vi "MainBancoEiettori.vi"() -> ()   [LabVIEW 2025]
uses:
  STATES_MACHINE.ctl
  <instrlib>/Bronkhorst FLOW-BUS/Public/Configure/Setpoint/Configure Setpoint (Direct).vi
  <instrlib>/Bronkhorst FLOW-BUS/Public/Data/Measure/Read Measure (Direct).vi
  <vilib>/Utility/file.llb/Write Delimited Spreadsheet (string).vi
  <vilib>/Utility/file.llb/Write Delimited Spreadsheet (DBL).vi
  <instrlib>/Bronkhorst FLOW-BUS/Bronkhorst FLOW-BUS.lvlib
panel:
  in  "Tab Control":enum32{"Main", "Debug"}(tab)
  in  "Sample Time":u16=100
  in  "Clear Graph":bool
  in  "Start Test Session":bool
  in  "stop":bool
  out "array":dbl[][](array[numeric]) format="%#_5g"
  out "Outlet  [mA]":dbl
  out "Secondary [mA]":dbl
  out "Primary [mA]":dbl
  out "Outlet [bar]":dbl
  out "Secondary [bar]":dbl
  out "Primary [bar]":dbl
  in  "Insert Case":bool
  in  "New test":bool
  out "Waveform Chart":T1(graph)
  out "Exit":bool
  out "_InsertCase":bool
  out "_NewTest":bool
  in  "VISA resource name 2":refnum<visa-resource-name>
  out "Fluid Name":string
  out "Capacity":sgl
  out "Capacity Unit":string
  out "Capacity Unit 2":string
  out "Capacity 2":sgl
  out "Fluid Name 2":string
  in  "VISA resource name 3":refnum<visa-resource-name>
  out "_StartSession":bool
  # "Current \nValve\n[mA]"
  # "Primary \nPressure\n[bar]"
  # "Secondary \nPressure\n[bar]"
  # "Outlet \nPressure\n[bar]"
  # "Mass Flow\nPrimary\nkg/min"
  # "Mass Flow\nSecondary\nkg/min"
  # "Actual Pressure Values"
  # "ms"
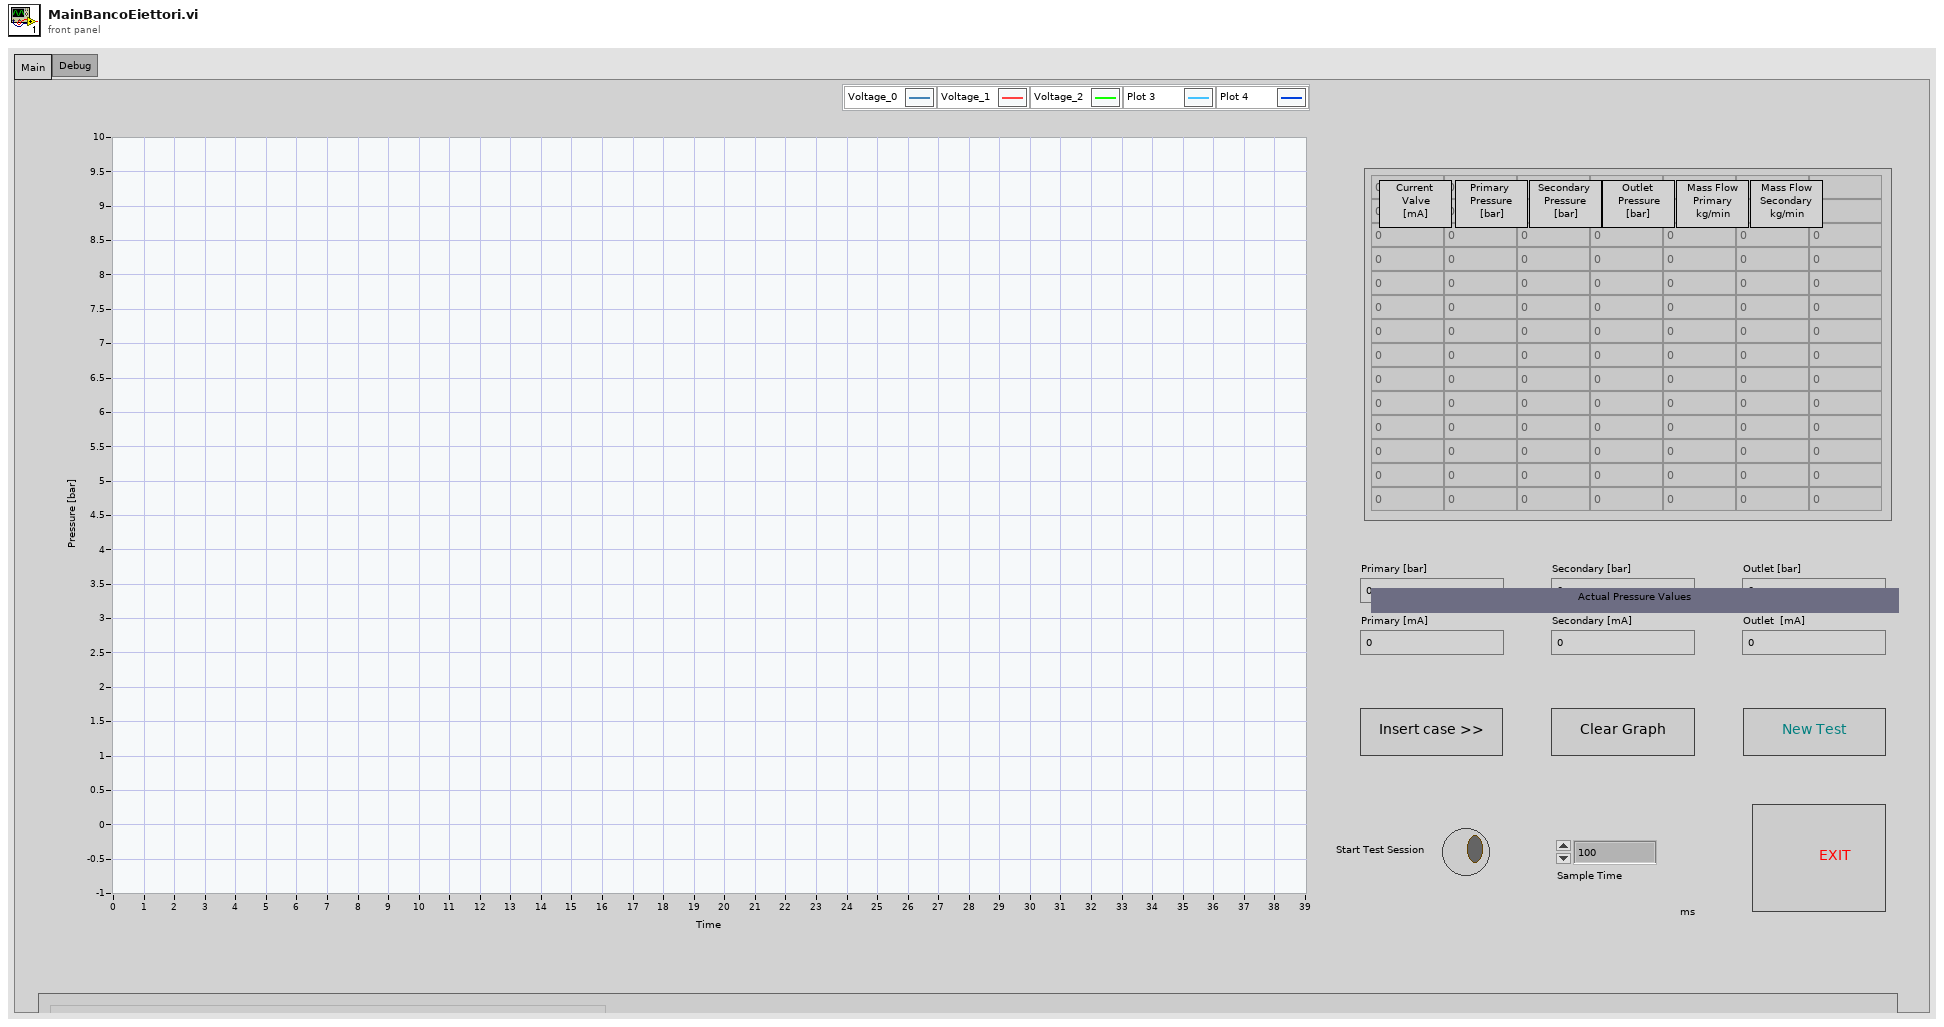
[diagram p1: front panel]
types:
  T1 = cluster{"Scalar":dbl, "Scalar":dbl, "Scalar":dbl, "number: 0 to 1":dbl, "number: 0 to 1":dbl}
  T2 = typedef "STATES_MACHINE.ctl" = enum16{"INIT", "TEST", "CLOSE"}
  T3 = cluster{"Scalar":dbl, "Scalar":dbl, "Scalar":dbl, "number: 0 to 1":dbl, "number: 0 to 1":dbl}[]
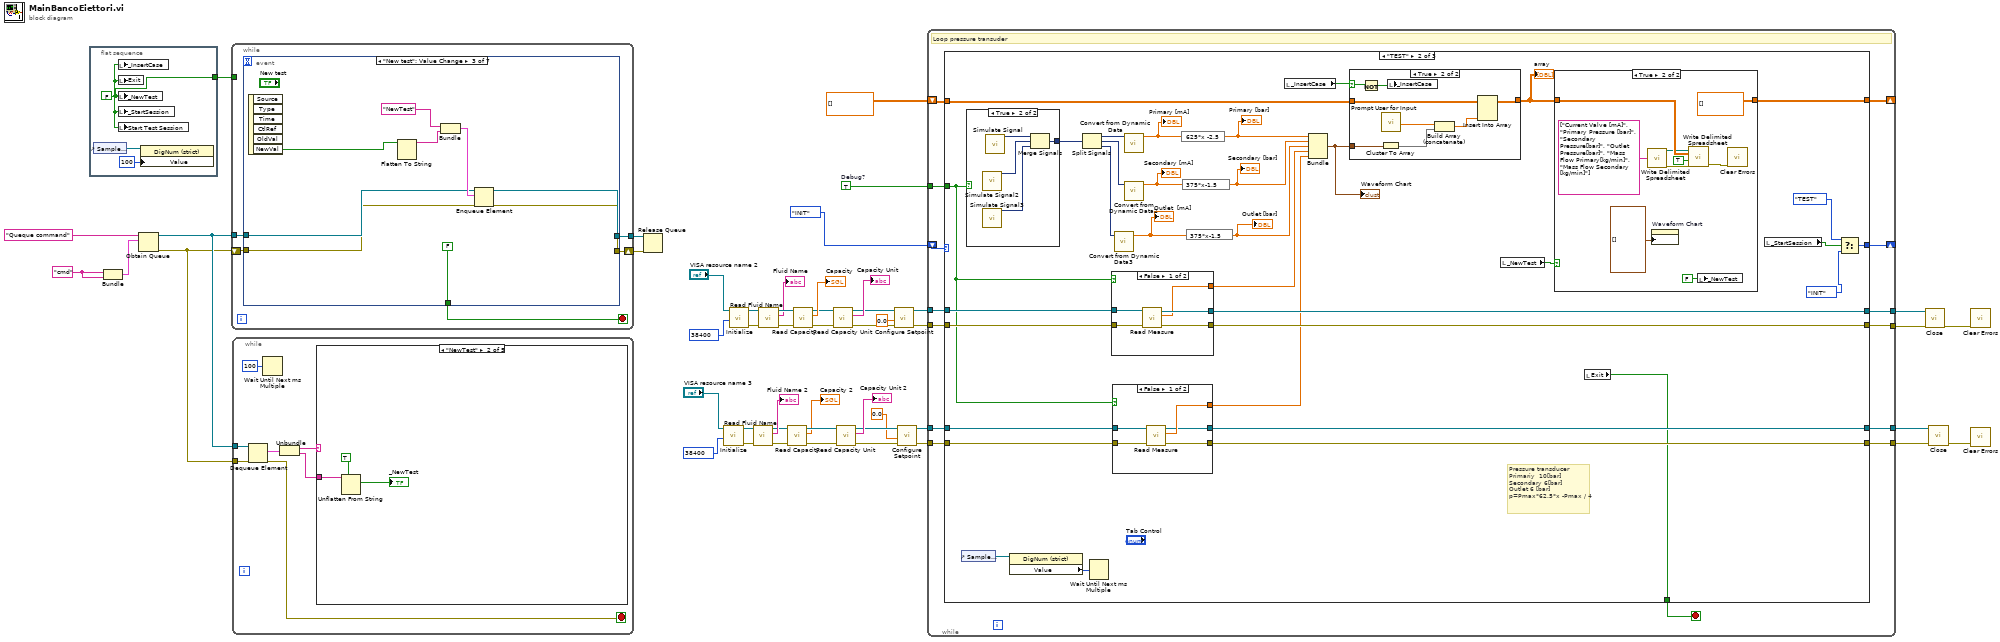
[diagram p0: block diagram]
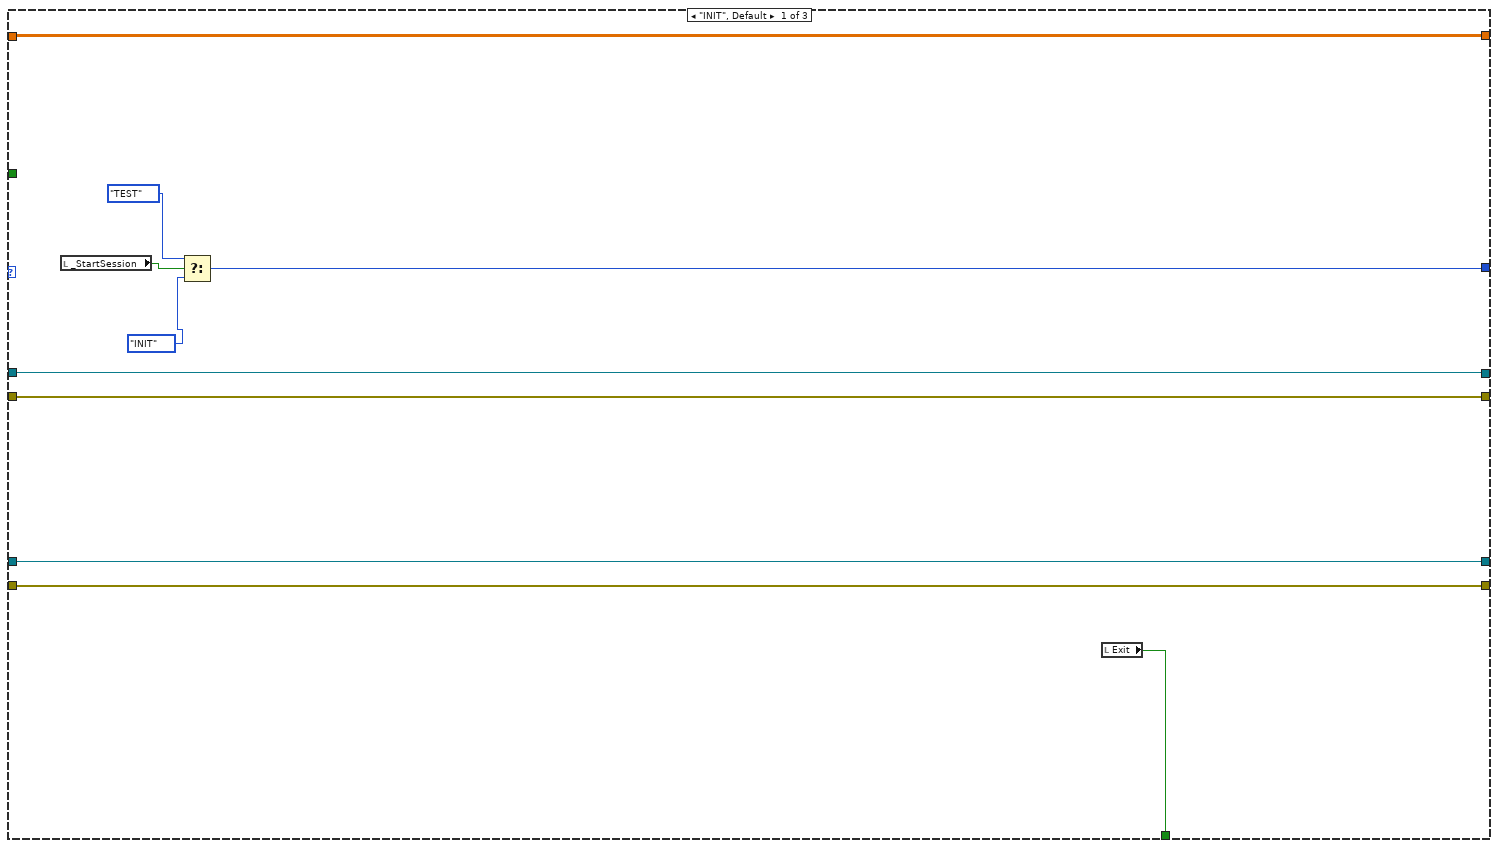
[diagram p2: hidden frame]
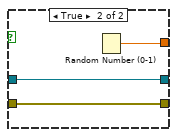
[diagram p3: hidden frame]
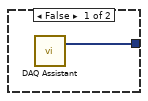
[diagram p4: hidden frame]
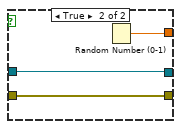
[diagram p7: hidden frame]
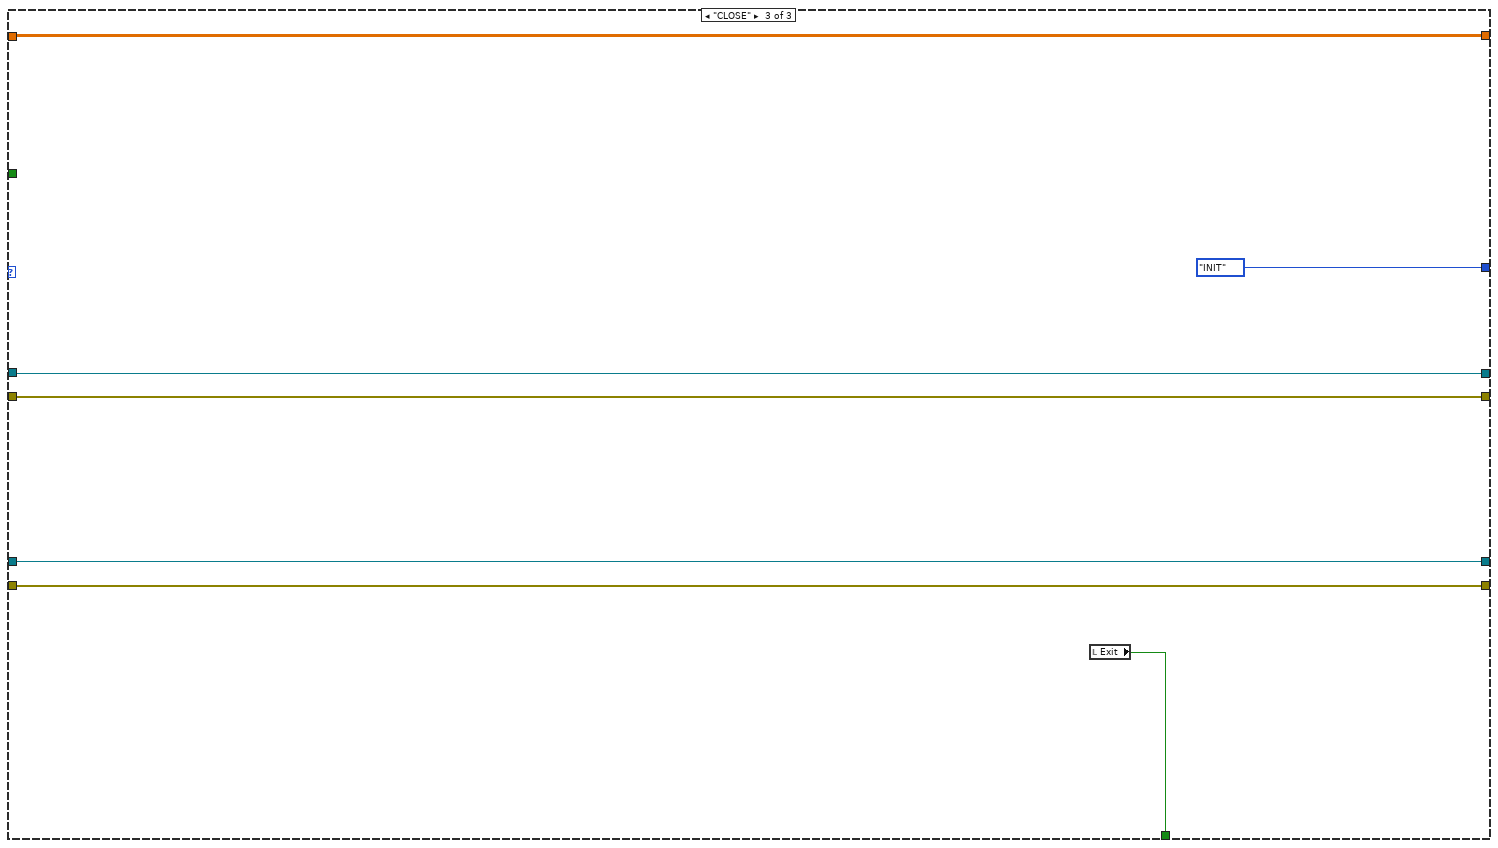
[diagram p8: hidden frame]
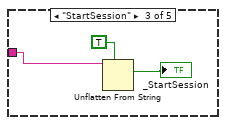
[diagram p10: hidden frame]
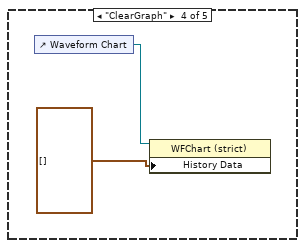
[diagram p11: hidden frame]
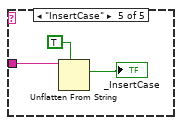
[diagram p12: hidden frame]
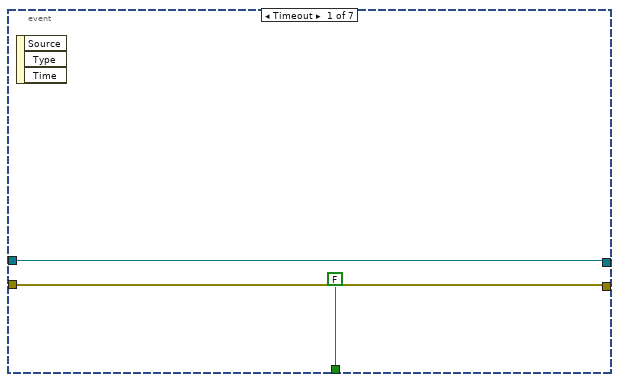
[diagram p13: hidden frame]
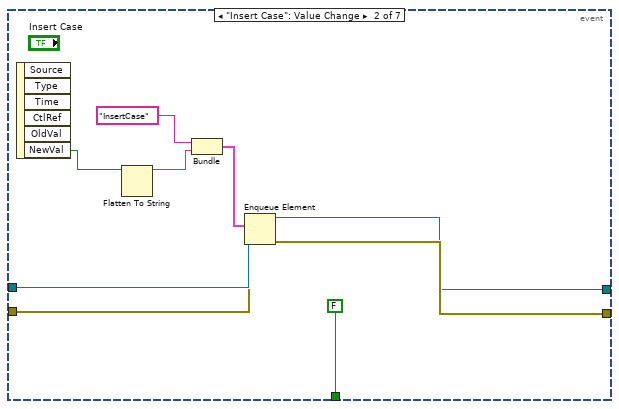
[diagram p14: hidden frame]
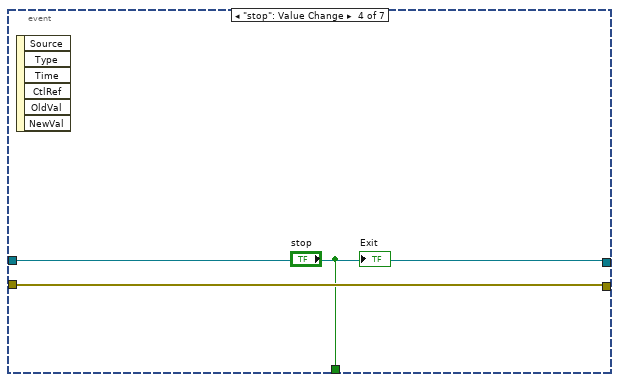
[diagram p15: hidden frame]
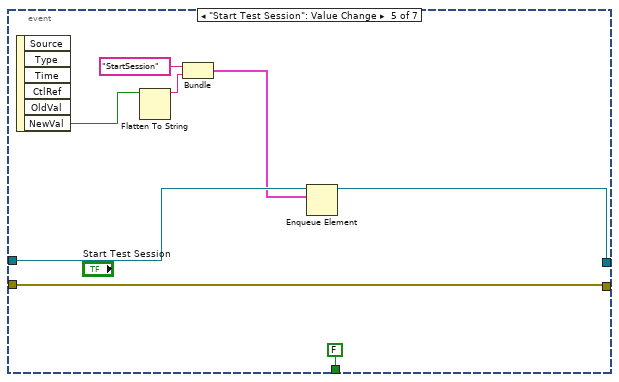
[diagram p16: hidden frame]
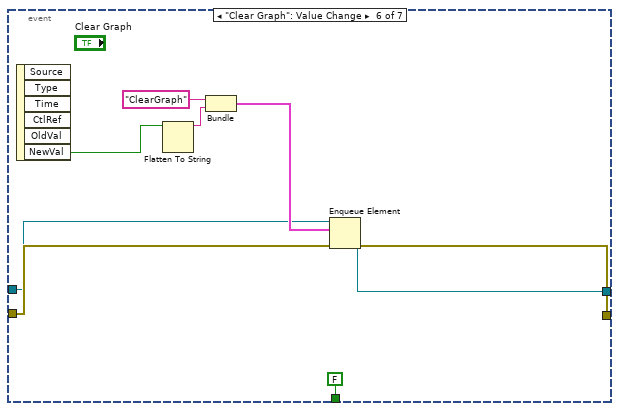
[diagram p17: hidden frame]
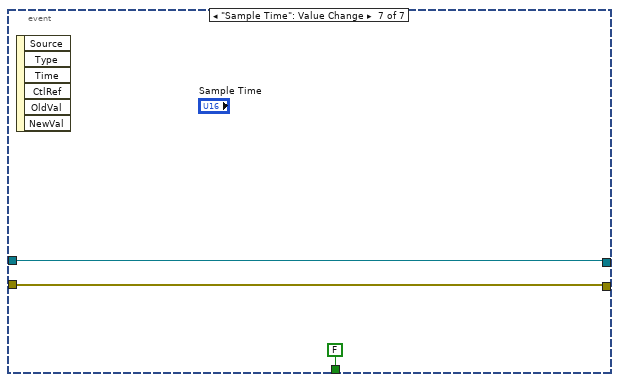
[diagram p18: hidden frame]
diagram:
  w13 = TRUE  # Debug?
  w27 = u32 38400 items=["9600"=9600, "19200"=19200, "38400"=38400, "57600"=57600, "115200"=115200, "230400"=230400, "460800"=460800] ("Baud Rate (38400)")
  w32 = u32 38400 items=["9600"=9600, "19200"=19200, "38400"=38400, "57600"=57600, "115200"=115200, "230400"=230400, "460800"=460800] ("Baud Rate (38400)")
  w42 = "cmd"
  n1 = flat-sequence {
    tunnel: [w52] -> w41
    frame #0 {
      w52 = FALSE ("_InsertCase 2")
      n2 = control-ref of="Sample Time"() -> (w51:refnum<vi>)
      n3 = local write "_InsertCase"(w52) -> ()
      n4 = local write "Exit"(w52) -> ()
      n5 = local write "_NewTest"(w52) -> ()
      n6 = local write "_StartSession"(w52) -> ()
      n7 = local write "Start Test Session"(w52) -> ()
      n8 = property class="DigNum (strict)"(reference=w51, "Value"=u16 100) -> ()  [unwired: 1 in, 2 out]
    }
  }
  n9 = Bundle(w42, w42) -> (w47:cluster{string, string})  [unwired: 1 in]
  n10 = Obtain Queue(name (unnamed)="Queque command", element data type=w47) -> (queue out=w44:refnum<queue>, error out=w43:errorcluster)  [unwired: 3 in, 1 out]
  n11 = while {
    tunnel: w44 -> [w57]
    shift-right: [w55] -> w45
    shift-left: w43 -> [w56]
    tunnel: [w54] -> w46
    tunnel: w41 -> [_]
    stop <- w53 stop-if-true
    n12 = event shown="[2] \"New test\": Value Change" {
      selector: _ -> [_ _ _ _ _ _ _]
      dyn-events: _ -> [_ _ _ _ _ _ _]
      timeout: _ -> [_ _ _ _ _ _ _]
      tunnel: w57 -> [w60 w69 w74 w81 w88 w92 w100]
      tunnel: w56 -> [w59 w68 w73 w80 w89 w95 w101]
      tunnel: [w59 w67 w71 w80 w89 w94 w101] -> w55
      tunnel: [w60 w66 w72 w81 w87 w93 w100] -> w54
      tunnel: [FALSE ("stop") FALSE ("stop") FALSE ("stop") "stop" FALSE ("stop") FALSE ("stop") FALSE ("stop")] -> w53
      event Timeout {
        n13 = event-data() -> ()  [unwired: 1 in, 3 out]
      }
      event "Insert Case": Value Change {
        n14 = event-data() -> ("NewVal"=w61:bool)  [unwired: 1 in, 5 out]
        n15 = Flatten To String(anything=w61) -> (data string=w64:string)  [unwired: 3 in, 2 out]
        n16 = Bundle("InsertCase", "data string"=w64) -> (w63:cluster{string, "data string":string})  [unwired: 1 in]
        n17 = Enqueue Element(queue=w69, element=w63, error in (no error)=w68) -> (queue out=w66:refnum<queue>, error out=w67:errorcluster)  [unwired: 1 in, 1 out]
      }
      event "New test": Value Change {
        n18 = event-data() -> ("NewVal"=w70:bool)  [unwired: 1 in, 5 out]
        n19 = Flatten To String(anything=w70) -> (data string=w76:string)  [unwired: 3 in, 2 out]
        n20 = Bundle("NewTest", "data string"=w76) -> (w75:cluster{string, "data string":string})  [unwired: 1 in]
        n21 = Enqueue Element(queue=w74, element=w75, error in (no error)=w73) -> (queue out=w72:refnum<queue>, error out=w71:errorcluster)  [unwired: 1 in, 1 out]
      }
      event "stop": Value Change {
        n22 = event-data() -> ()  [unwired: 1 in, 6 out]
        "Exit" <- "stop"
      }
      event "Start Test Session": Value Change {
        n23 = event-data() -> ("NewVal"=w85:bool)  [unwired: 1 in, 5 out]
        n24 = Flatten To String(anything=w85) -> (data string=w84:string)  [unwired: 3 in, 2 out]
        n25 = Bundle("StartSession", "data string"=w84) -> (w83:cluster{string, "data string":string})  [unwired: 1 in]
        n26 = Enqueue Element(queue=w88, element=w83) -> (queue out=w87:refnum<queue>)  [unwired: 2 in, 2 out]
      }
      event "Clear Graph": Value Change {
        n27 = event-data() -> ("NewVal"=w91:bool)  [unwired: 1 in, 5 out]
        n28 = Flatten To String(anything=w91) -> (data string=w97:string)  [unwired: 3 in, 2 out]
        n29 = Bundle("ClearGraph", "data string"=w97) -> (w96:cluster{string, "data string":string})  [unwired: 1 in]
        n30 = Enqueue Element(queue=w92, element=w96, error in (no error)=w95) -> (queue out=w93:refnum<queue>, error out=w94:errorcluster)  [unwired: 1 in, 1 out]
      }
      event "Sample Time": Value Change {
        n31 = event-data() -> ()  [unwired: 1 in, 6 out]
      }
    }
  }
  n32 = while {
    tunnel: w44 -> [w107]
    tunnel: w43 -> [w106]
    stop <- w102 stop-if-true
    n33 = Dequeue Element(queue=w107, error in (no error)=w106) -> (element=w105:cluster{string, string}, error out=w102:errorcluster)  [unwired: 1 in, 2 out]
    n34 = Wait Until Next ms Multiple(millisecond multiple=u32 100) -> ()  [unwired: 1 out]
    n35 = Unbundle(w105) -> (w104:string, w103:string)
    n36 = case shown="\"NewTest\"" w104 {
      tunnel: w103 -> [_ w110 w112 _ w119]
      frame "False", Default {
      }
      frame "NewTest" {
        n37 = Unflatten From String(type=TRUE, binary string=w110) -> (value=→"_NewTest":bool)  [unwired: 3 in, 2 out]
      }
      frame "StartSession" {
        n38 = Unflatten From String(type=TRUE, binary string=w112) -> (value=→"_StartSession":bool)  [unwired: 3 in, 2 out]
      }
      frame "ClearGraph" {
        n39 = control-ref of="Waveform Chart"() -> (w115:refnum<vi>)
        n40 = property on="Property Node" class="WFChart (strict)"(reference=w115, "History Data"=T3 []) -> ()  [unwired: 1 in, 2 out]
      }
      frame "InsertCase" {
        n41 = Unflatten From String(type=TRUE, binary string=w119) -> (value=→"_InsertCase":bool)  [unwired: 3 in, 2 out]
      }
    }
  }
  n42 = Release Queue(queue=w46, error in (no error)=w45) -> ()  [unwired: 1 in, 3 out]
  n43 = call <instrlib>:"Initialize.vi"("Baud Rate (38400)"=w27, "VISA resource name"="VISA resource name 3") -> ("error out"=w29:errorcluster, "VISA resource name out"=w28:refnum<visa-resource-name>)  [unwired: 8 in]
  n44 = call <instrlib>:"Initialize.vi"("Baud Rate (38400)"=w32, "VISA resource name"="VISA resource name 2") -> ("error out"=w30:errorcluster, "VISA resource name out"=w31:refnum<visa-resource-name>)  [unwired: 8 in]
  n45 = call <instrlib>:"Read Fluid Name.vi"("error in (no error)"=w29, "VISA resource name"=w28) -> ("error out"=w23:errorcluster, "Fluid Name"=→"Fluid Name 2":string, "VISA resource name out"=w24:refnum<visa-resource-name>)  [unwired: 7 in]
  n46 = call <instrlib>:"Read Fluid Name.vi"("error in (no error)"=w30, "VISA resource name"=w31) -> ("error out"=w36:errorcluster, "Fluid Name"=→"Fluid Name":string, "VISA resource name out"=w35:refnum<visa-resource-name>)  [unwired: 7 in]
  n47 = call <instrlib>:"Read Capacity.vi"("error in (no error)"=w23, "VISA resource name"=w24) -> ("error out"=w21:errorcluster, "Capacity"=→"Capacity 2":sgl, "VISA resource name out"=w22:refnum<visa-resource-name>)  [unwired: 7 in]
  n48 = call <instrlib>:"Read Capacity.vi"("error in (no error)"=w36, "VISA resource name"=w35) -> ("error out"=w38:errorcluster, "Capacity"=→"Capacity":sgl, "VISA resource name out"=w37:refnum<visa-resource-name>)  [unwired: 7 in]
  n49 = call <instrlib>:"Read Capacity Unit.vi"("error in (no error)"=w38, "VISA resource name"=w37) -> ("error out"=w3:errorcluster, "Capacity Unit"=→"Capacity Unit":string, "VISA resource name out"=w5:refnum<visa-resource-name>)  [unwired: 7 in]
  n50 = call <instrlib>:"Read Capacity Unit.vi"("error in (no error)"=w21, "VISA resource name"=w22) -> ("error out"=w8:errorcluster, "Capacity Unit"=→"Capacity Unit 2":string, "VISA resource name out"=w18:refnum<visa-resource-name>)  [unwired: 7 in]
  n51 = call-poly <instrlib>:"Configure Setpoint.vi"("error in (no error)"=w3, "Setpoint Direct (0)"=sgl 0.0, "VISA resource name"=w5) -> ("error out"=w2:errorcluster, "VISA resource name out"=w4:refnum<visa-resource-name>)  [unwired: 7 in]
  n52 = call-poly <instrlib>:"Configure Setpoint.vi"("error in (no error)"=w8, "Setpoint Direct (0)"=sgl 0.0, "VISA resource name"=w18) -> ("error out"=w7:errorcluster, "VISA resource name out"=w9:refnum<visa-resource-name>)  [unwired: 7 in]
  n53 = while {
    shift-right: [w131] -> _
    shift-left: dbl[][] [] ("array") -> [w132]
    tunnel: w4 -> [w129]
    tunnel: w9 -> [w125]
    tunnel: w7 -> [w126]
    tunnel: w2 -> [w130]
    tunnel: [w127] -> w17
    tunnel: [w123] -> w16
    tunnel: [w124] -> w15
    tunnel: [w128] -> w14
    tunnel: w13 -> [w122]
    shift-right: [w120] -> _
    shift-left: STATES_MACHINE."INIT" ("Enum") -> [w121]
    stop <- w133 stop-if-true
    # "Loop pressure transuder"
    n54 = case shown="\"TEST\"" w121 {
      tunnel: [w139 w150 w224] -> w133
      tunnel: w132 -> [w134 w174 w218]
      tunnel: [w134 w167 w218] -> w131
      tunnel: w130 -> [w137 w163 w221]
      tunnel: w129 -> [w138 w162 w222]
      tunnel: [w137 w161 w221] -> w128
      tunnel: [w138 w160 w222] -> w127
      tunnel: w126 -> [w135 w157 w219]
      tunnel: w125 -> [w136 w156 w220]
      tunnel: [w135 w155 w219] -> w124
      tunnel: [w136 w153 w220] -> w123
      tunnel: w122 -> [_ w152 _]
      tunnel: [w140 w146 STATES_MACHINE."INIT" ("Enum")] -> w120
      frame "INIT", Default {
        n55 = local read "_StartSession"() -> (w143:bool)
        n56 = Select(t=STATES_MACHINE."TEST" ("Enum"), s=w143, f=STATES_MACHINE."INIT" ("Enum")) -> (s? t:f=w140:T2)
        n57 = local read "Exit"() -> (w139:bool)
      }
      frame "TEST" {
        # "Pressure transducer \nPrimariy  10[bar]\nSecondary 6[bar]\nOutlet 6 [bar]\np=Pmax*62.5*x -Pmax / 4"
        n58 = control-ref of="Sample Time"() -> (w145:refnum<vi>)
        n59 = case shown="True" w152 {
          tunnel: [w186 w187] -> w166
          frame False {
            n60 = call "DAQ Assistant"() -> ("data"=w186:dynamicdata)  [unwired: 17 in, 2 out]
          }
          frame True {
            n61 = call "Simulate Signal2"() -> ("Sine"=w189:dynamicdata)  [unwired: 14 in, 1 out]
            n62 = call "Simulate Signal3"() -> ("Sine"=w190:dynamicdata)  [unwired: 14 in, 1 out]
            n63 = call "Simulate Signal"() -> ("Sine"=w188:dynamicdata)  [unwired: 14 in, 1 out]
            n64 = Merge Signals(w188, w189, w190) -> (w187:dynamicdata)
          }
        }
        n65 = property class="DigNum (strict)"(reference=w145) -> ("Value"=w144:u16)  [unwired: 1 in, 2 out]
        n66 = Split Signals(w166) -> (w177:dynamicdata, w176:dynamicdata, w175:dynamicdata)  [unwired: 3 in]
        n67 = Wait Until Next ms Multiple(millisecond multiple=w144) -> ()  [unwired: 1 out]
        n68 = case shown="False" w152 {
          tunnel: w163 -> [w214 w216]
          tunnel: w162 -> [w213 w217]
          tunnel: [w212 w216] -> w161
          tunnel: [w211 w217] -> w160
          tunnel: [w210 w215] -> w158
          frame False {
            n69 = call-poly <instrlib>:"Read Measure.vi"("error in (no error)"=w214, "VISA resource name"=w213) -> ("error out"=w212:errorcluster, "Measure Direct"=w210:sgl, "VISA resource name out"=w211:refnum<visa-resource-name>)  [unwired: 7 in]
          }
          frame True {
            n70 = Random Number (0-1)() -> (number: 0 to 1=w215:dbl)
          }
        }
        n71 = case shown="False" w152 {
          tunnel: w157 -> [w182 w184]
          tunnel: w156 -> [w181 w185]
          tunnel: [w180 w184] -> w155
          tunnel: [w179 w183] -> w154
          tunnel: [w178 w185] -> w153
          frame False {
            n72 = call-poly <instrlib>:"Read Measure.vi"("error in (no error)"=w182, "VISA resource name"=w181) -> ("error out"=w180:errorcluster, "Measure Direct"=w179:sgl, "VISA resource name out"=w178:refnum<visa-resource-name>)  [unwired: 7 in]
          }
          frame True {
            n73 = Random Number (0-1)() -> (number: 0 to 1=w183:dbl)
          }
        }
        n74 = call "Convert from Dynamic Data3"("Dynamic Data Type"=w175) -> ("Scalar"=w171:dbl)  [unwired: 3 in]
        "Outlet  [mA]" <- w171
        n75 = call "Convert from Dynamic Data"("Dynamic Data Type"=w177) -> ("Scalar"=w173:dbl)  [unwired: 3 in]
        "Primary [mA]" <- w173
        n76 = call "Convert from Dynamic Data2"("Dynamic Data Type"=w176) -> ("Scalar"=w172:dbl)  [unwired: 3 in]
        "Secondary [mA]" <- w172
        n77 = expression code="625*x -2.5"(w173) -> (w151:dbl)
        "Primary [bar]" <- w151
        n78 = expression code="375*x-1.5"(w172) -> (w165:dbl)
        "Secondary [bar]" <- w165
        n79 = expression code="375*x-1.5"(w171) -> (w164:dbl)
        "Outlet [bar]" <- w164
        n80 = local read "_InsertCase"() -> (w170:bool)
        n81 = Bundle("Scalar"=w151, "Scalar"=w165, "Scalar"=w164, "number: 0 to 1"=w158, "number: 0 to 1"=w154) -> (w159:T1)  [unwired: 1 in]
        "Waveform Chart" <- w159
        n82 = case shown="True" w170 {
          selector: w170 -> [_ w205]
          tunnel: [w201 w209] -> w168
          tunnel: w174 -> [w201 w206]
          tunnel: w159 -> [_ w203]
          frame False {
          }
          frame True {
            n83 = Not(x=w205) -> (.not. x?=w204:bool)
            n84 = Cluster To Array(cluster=w203) -> (array=w202:dbl[])
            n85 = call "Prompt User for Input"() -> ("Current"=w207:dbl)  [unwired: 17 in, 2 out]
            n86 = local write "_InsertCase"(w204) -> ()
            n87 = Build Array (concatenate)(w207, w202) -> (w208:dbl[])
            n88 = Insert Into Array(array=w206, new element=w208) -> (w209:dbl[][])  [unwired: 2 in]
          }
        }
        "array" <- w168
        n89 = local read "_NewTest"() -> (w169:bool)
        n90 = case shown="True" w169 {
          tunnel: w168 -> [w191 w199]
          tunnel: [w191 dbl[][] [] ("array")] -> w167
          frame False {
          }
          frame True {
            n91 = call-poly <vilib>:"Write Delimited Spreadsheet.vi"("1D data"=string[] ["Current Valve [mA]", "Primary Pressure [bar]", "Secondary Pressure[bar]", "Outlet Pressure[bar]", "Mass Flow Primary[kg/min]", "Mass Flow Secondary [kg/min]"]) -> ("new file path (Not A Path if cancelled)"=w193:path, "error out"=w194:errorcluster)  [unwired: 13 in]
            n92 = property on="Waveform Chart" class="WFChart (strict)"("History Data"=T3 []) -> ()  [unwired: 2 in, 2 out]
            n93 = call-poly <vilib>:"Write Delimited Spreadsheet.vi"("file path (dialog if empty)"=w193, "2D data"=w199, "append to file? (new file:F)"=TRUE, "error in (no error)"=w194) -> ("error out"=w197:errorcluster)  [unwired: 10 in, 1 out]
            n94 = local write "_NewTest"(FALSE ("_NewTest")) -> ()
            n95 = call <vilib>:"Clear Errors.vi"("error in (no error)"=w197) -> ()  [unwired: 5 in, 2 out]
          }
        }
        n96 = local read "Exit"() -> (w150:bool)
        n97 = local read "_StartSession"() -> (w149:bool)
        n98 = Select(t=STATES_MACHINE."TEST" ("Enum"), s=w149, f=STATES_MACHINE."INIT" ("Enum")) -> (s? t:f=w146:T2)
      }
      frame "CLOSE" {
        n99 = local read "Exit"() -> (w224:bool)
      }
    }
  }
  n100 = call <instrlib>:"Close.vi"("error in (no error)"=w14, "VISA resource name"=w17) -> ("error out"=w12:errorcluster)  [unwired: 9 in]
  n101 = call <instrlib>:"Close.vi"("error in (no error)"=w15, "VISA resource name"=w16) -> ("error out"=w11:errorcluster)  [unwired: 9 in]
  n102 = call <vilib>:"Clear Errors.vi"("error in (no error)"=w12) -> ()  [unwired: 5 in, 2 out]
  n103 = call <vilib>:"Clear Errors.vi"("error in (no error)"=w11) -> ()  [unwired: 5 in, 2 out]
